vi "CloseConfigFP.vi"(8 "error in (no error)":errorcluster, 10 "Ancestor":string, 11 "reference in":refnum<class "ViPER.lvclass">) -> (0 "error out":errorcluster, 3 "reference out":refnum<class "ViPER.lvclass">)   [LabVIEW 2022 SP3, in "ViPER.lvlib" / "ViPER.lvclass"]
doc: "### BSD License (http://www.opensource.org/licenses/bsd-license.php) Begin ###\n\nCopyright (c) 2018 Kurt Friday www.medulla.net\n\nAll rights reserved.\n\nRedistribution and use in source and binary forms, with or without\nmodification, are permitted provided that the following conditions are met:\n\n * Redistributions of source code must retain the above copyright\n notice, this list of conditions and the following disclaimer.\n\n * Redistributions in binary form must reproduce the above copyright\n notice, this list of conditions and the following disclaimer in the\n documentation and/or other materials provided with the distribution.\n\n * Neither the name of the <organization> nor the\n names of its contributors may be used to endorse or promote products\n derived from this software without specific prior written permission.\n\nTHIS SOFTWARE IS PROVIDED BY THE COPYRIGHT HOLDERS AND CONTRIBUTORS \"AS IS\" AND\nANY EXPRESS OR IMPLIED WARRANTIES, INCLUDING, BUT NOT LIMITED TO, THE IMPLIED\nWARRANTIES OF MERCHANTABILITY AND FITNESS FOR A PARTICULAR PURPOSE ARE\nDISCLAIMED. IN NO EVENT SHALL <COPYRIGHT HOLDER> BE LIABLE FOR ANY\nDIRECT, INDIRECT, INCIDENTAL, SPECIAL, EXEMPLARY, OR CONSEQUENTIAL DAMAGES\n(INCLUDING, BUT NOT LIMITED TO, PROCUREMENT OF SUBSTITUTE GOODS OR SERVICES;\nLOSS OF USE, DATA, OR PROFITS; OR BUSINESS INTERRUPTION) HOWEVER CAUSED AND\nON ANY THEORY OF LIABILITY, WHETHER IN CONTRACT, STRICT LIABILITY, OR TORT\n(INCLUDING NEGLIGENCE OR OTHERWISE) ARISING IN ANY WAY OUT OF THE USE OF THIS\nSOFTWARE, EVEN IF ADVISED OF THE POSSIBILITY OF SUCH DAMAGE."
uses:
  ViPER.lvclass
panel:
  # "### BSD License (http://www.opensource.org/licenses/bsd-license.php) Begin ###\n\nCopyright (c) 2018  Kurt Friday www.medulla.net\n\nAll rights reserved.\n\nRedistribution and use in source and binary forms, with or without\nmodification, are permitted provided that the following conditions are met:\n\n    * Redistributions of source code must retain the above copyright\n      notice, this list of conditions and the following disclaimer.\n\n    * Redistributions in binary form must reproduce the above copyright\n      notice, this list of conditions and the following disclaimer in the\n      documentation and/or other materials provided with the distribution.\n\n    * Neither the name of the <organization> nor the\n      names of its contributors may be used to endorse or promote products\n      derived from this software without specific prior written permission.\n\nTHIS SOFTWARE IS PROVIDED BY THE COPYRIGHT HOLDERS AND CONTRIBUTORS \"AS IS\" AND\nANY EXPRESS OR IMPLIED WARRANTIES, INCLUDING, BUT NOT LIMITED TO, THE IMPLIED\nWARRANTIES OF MERCHANTABILITY AND FITNESS FOR A PARTICULAR PURPOSE ARE\nDISCLAIMED. IN NO EVENT SHALL <COPYRIGHT HOLDER> BE LIABLE FOR ANY\nDIRECT, INDIRECT, INCIDENTAL, SPECIAL, EXEMPLARY, OR CONSEQUENTIAL DAMAGES\n(INCLUDING, BUT NOT LIMITED TO, PROCUREMENT OF SUBSTITUTE GOODS OR SERVICES;\nLOSS OF USE, DATA, OR PROFITS; OR BUSINESS INTERRUPTION) HOWEVER CAUSED AND\nON ANY THEORY OF LIABILITY, WHETHER IN CONTRACT, STRICT LIABILITY, OR TORT\n(INCLUDING NEGLIGENCE OR OTHERWISE) ARISING IN ANY WAY OUT OF THE USE OF THIS\nSOFTWARE, EVEN IF ADVISED OF THE POSSIBILITY OF SUCH DAMAGE."
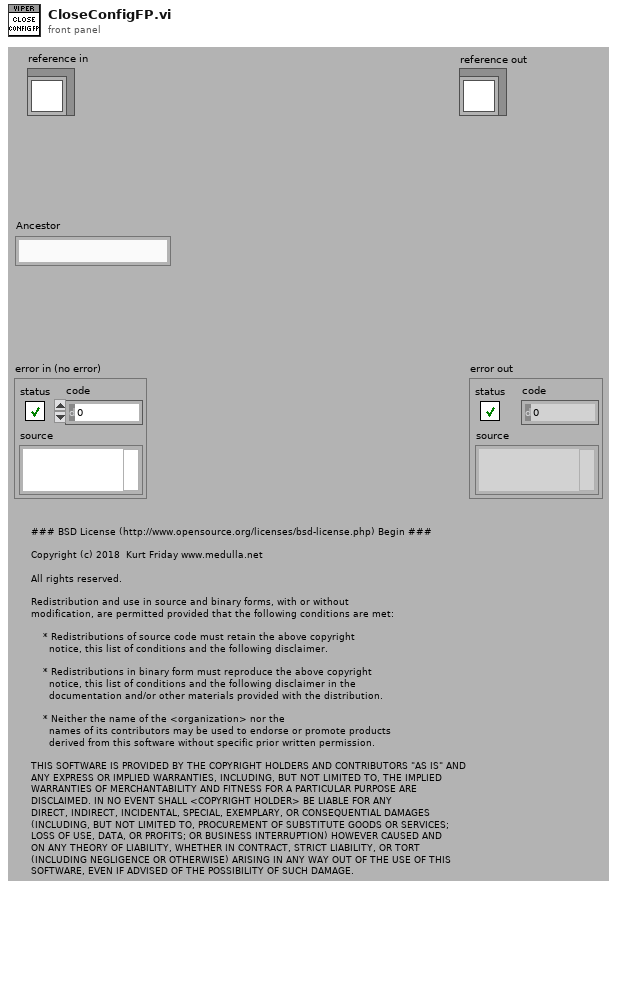
[diagram p1: front panel]
types:
  T1 = typedef "ViPER.lvlib/ViPER.lvclass/Details.ctl" = cluster{"Name":string, "Class":string}
  T2 = typedef "ViPER.lvlib/ViPER.lvclass/ObjectAttributes.ctl" = cluster{"Object":T3, "Ancestors":T5[], "Config":T6, "Init_OK":bool, "Hierachy":string[], "PPL?":bool[], "SFP_Open":bool[], "Config_SFP_Open":bool[], "SoftFP_event":refnum<user-event>[], "ConfigFP_event":refnum<user-event>[], "SoftFP_Shutdown_Notifier":refnum<notifier>[], "ConfigFP_Shutdown_Notifier":refnum<notifier>[]}
  T3 = typedef "ViPER.lvlib/ViPER.lvclass/ObjectDefinition.ctl" = cluster{"Name":string, "Ancestors":T4[]}
  T4 = typedef "ViPER.lvlib/ViPER.lvclass/Ancestor.ctl" = cluster{"Class":string, "Config":string, "Objects":string[]}
  T5 = typedef "ViPER.lvlib/ViPER.lvclass/ObjectLayers.ctl" = cluster{"Ancestor":string, "Objects":refnum<class "ViPER.lvclass">[], "Object_Names":string[], "Owned":bool[]}
  T6 = typedef "ViPER.lvlib/ViPER.lvclass/Config.ctl" = cluster{"default":string}
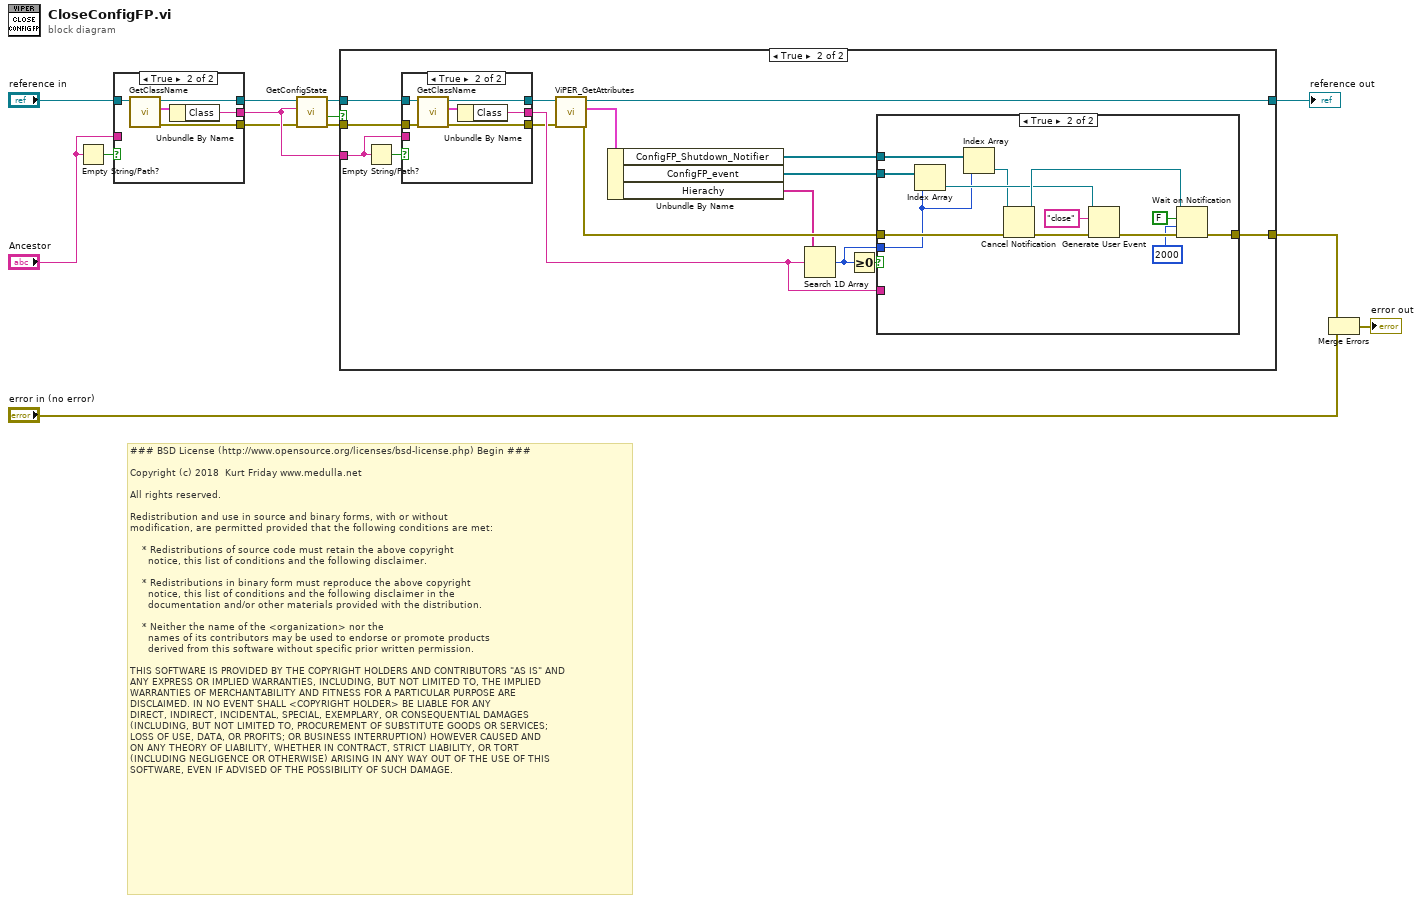
[diagram p0: block diagram]
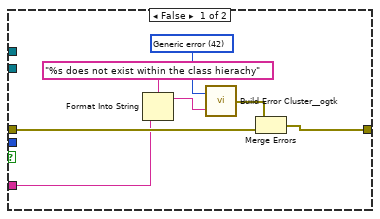
[diagram p5: hidden frame]
diagram:
  # "### BSD License (http://www.opensource.org/licenses/bsd-license.php) Begin ###\n\nCopyright (c) 2018  Kurt Friday www.medulla.net\n\nAll rights reserved.\n\nRedistribution and use in source and binary forms, with or without\nmodification, are permitted provided that the following conditions are met:\n\n    * Redistributions of source code must retain the above copyright\n      notice, this list of conditions and the following disclaimer.\n\n    * Redistributions in binary form must reproduce the above copyright\n      notice, this list of conditions and the following disclaimer in the\n      documentation and/or other materials provided with the distribution.\n\n    * Neither the name of the <organization> nor the\n      names of its contributors may be used to endorse or promote products\n      derived from this software without specific prior written permission.\n\nTHIS SOFTWARE IS PROVIDED BY THE COPYRIGHT HOLDERS AND CONTRIBUTORS \"AS IS\" AND\nANY EXPRESS OR IMPLIED WARRANTIES, INCLUDING, BUT NOT LIMITED TO, THE IMPLIED\nWARRANTIES OF MERCHANTABILITY AND FITNESS FOR A PARTICULAR PURPOSE ARE\nDISCLAIMED. IN NO EVENT SHALL <COPYRIGHT HOLDER> BE LIABLE FOR ANY\nDIRECT, INDIRECT, INCIDENTAL, SPECIAL, EXEMPLARY, OR CONSEQUENTIAL DAMAGES\n(INCLUDING, BUT NOT LIMITED TO, PROCUREMENT OF SUBSTITUTE GOODS OR SERVICES;\nLOSS OF USE, DATA, OR PROFITS; OR BUSINESS INTERRUPTION) HOWEVER CAUSED AND\nON ANY THEORY OF LIABILITY, WHETHER IN CONTRACT, STRICT LIABILITY, OR TORT\n(INCLUDING NEGLIGENCE OR OTHERWISE) ARISING IN ANY WAY OUT OF THE USE OF THIS\nSOFTWARE, EVEN IF ADVISED OF THE POSSIBILITY OF SUCH DAMAGE."
  n1 = Empty String/Path?(string/path="Ancestor") -> (empty?=w6:bool)
  n2 = case shown="True" w6 {
    tunnel: [_ w20] -> w1
    tunnel: "reference in" -> [w15 w19]
    tunnel: [w15 w18] -> w4
    tunnel: "Ancestor" -> [w14 _]
    tunnel: [w14 w16] -> w2
    frame False {
    }
    frame True {
      n3 = call "GetClassName.vi"("reference in"=w19) -> ("error out"=w20:errorcluster, "Details"=w17:T1, "reference out"=w18:refnum<class "ViPER.lvclass">)  [unwired: 8 in]
      n4 = Unbundle By Name(w17) -> ("Class"=w16:string)
    }
  }
  n5 = call-dynamic "GetConfigState.vi"("error in (no error)"=w1, "Ancestor"=w2, "reference in"=w4) -> ("error out"=w10:errorcluster, "config_open"=w9:bool, "reference out"=w11:refnum<class "ViPER.lvclass">)  [unwired: 6 in]
  n6 = case shown="True" w9 {
    tunnel: [w21 w36] -> w7
    tunnel: [w22 w35] -> w8
    tunnel: w11 -> [w22 w29]
    tunnel: w10 -> [w21 w27]
    tunnel: w2 -> [_ w24]
    frame False {
    }
    frame True {
      n7 = Empty String/Path?(string/path=w24) -> (empty?=w26:bool)
      n8 = case shown="True" w26 {
        tunnel: w27 -> [w39 w47]
        tunnel: [w39 w46] -> w23
        tunnel: w29 -> [w41 w45]
        tunnel: [w41 w44] -> w28
        tunnel: w24 -> [w40 _]
        tunnel: [w40 w42] -> w25
        frame False {
        }
        frame True {
          n9 = call "GetClassName.vi"("error in (no error)"=w47, "reference in"=w45) -> ("error out"=w46:errorcluster, "Details"=w43:T1, "reference out"=w44:refnum<class "ViPER.lvclass">)  [unwired: 7 in]
          n10 = Unbundle By Name(w43) -> ("Class"=w42:string)
        }
      }
      n11 = call "ViPER_GetAttributes.vi"("error in (no error)"=w23, "reference in"=w28) -> ("error out"=w34:errorcluster, "Data"=w38:T2, "reference out"=w35:refnum<class "ViPER.lvclass">)  [unwired: 6 in, 1 out]
      n12 = Unbundle By Name(w38) -> ("ConfigFP_Shutdown_Notifier"=w33:refnum<notifier>[], "ConfigFP_event"=w37:refnum<user-event>[], "Hierachy"=w32:string[])
      n13 = Search 1D Array(1D array=w32, element=w25) -> (index of element=w30:i32)  [unwired: 1 in]
      n14 = Greater Or Equal To 0?(x=w30) -> (x >= 0?=w31:bool)
      n15 = case shown="True" w31 {
        tunnel: w37 -> [_ w59]
        tunnel: [w49 w67] -> w36
        tunnel: w34 -> [w50 w66]
        tunnel: w33 -> [_ w57]
        tunnel: w30 -> [_ w56]
        tunnel: w25 -> [w48 _]
        frame False {
          w51 = 42 items=["No error", "Argument error", "Memory is full", "Out of zone", "End of file", "File already open", "Generic file I/O error", "File not found", "File permission error", "Disk is full", "Duplicate path", "Too many files open", "System feature not enabled", "Resource file not found", "Cannot add resource", "Resource not found", "Image not found", "Image memory error", "Pen does not exist", "Config type invalid", "Config token not found", "Config parse error", "Config memory error", "Bad external code format", "Bad external code offset", "External code not present", "Null window", "Destroy window error", "Null menu", "Print aborted", "Bad print record", "Print driver error", "Windows error during printing", "Memory error during printing", "Print dialog error", "Generic print error", "Invalid device refnum", "Device not found", "Device parameter error", "Device unit error", "Cannot open device", "Device call aborted", "Generic error", "Cancelled by user", "Object ID too low", "Object ID too high", "Object not in heap", "Unknown heap", "Unknown object (invalid DefProc)", "Unknown object (DefProc not in table)", "Message out of range", "Invalid (null) method", "Unknown message", "Manager call not supported", "Bad address", "Network operation in progress", "Network operation timed out", "Connection is busy", "Network attribute not supported", "Network error", "Address in use", "System out of memory", "Connection aborted", "Connection refused", "Not connected", "Already connected", "Connection closed", "Initialization error (interapplication manager)", "Bad occurrence", "Wait on unbound occurrence handler", "Occurrence queue overflow", "Datalog type conflict", "Unused", "Unrecognized type (interapplication manager)", "Memory corrupt", "Failed to make temporary DLL", "Old CIN version", "Drag socket not found", "Failed to load drop-object", "Failed to register OLE object", "Failed to release OLE object", "Format specifier type mismatch", "Unknown format specifier", "Too few format specifiers", "Too many format specifiers", "Scan failed", "Newer CIN version", "Error converting to variant", "Runtime menu error", "Password tampered", "Variant attribute not found", "Incompatible variant data type", "Event data is not available", "Event Store is not present", "Occurrence is not found", "Event Queue is not created", "Event info is not available", "Refnum passed is NULL", "Error retrieving Class GUID", "Error retrieving CoClass GUID", "Error retrieving TypeLib GUID.", "Bad built application magic bytes.", "Specific driver is different from the specific driver associated with the Logical Name.", "There is no session opened to the class driver.", "Max Error", "MAX - Error with config objects", "MAX - Error loading configuration", "MAX - Group not supported"]
          n16 = Format Into String(format string="%s does not exist within the class hierachy", w48) -> (resulting string=w54:string)  [unwired: 2 in, 1 out]
          n17 = call <userlib>:"Build Error Cluster__ogtk.vi"("String to Prepend to source (\"\")"=w54, "code"=w51) -> ("error out"=w52:errorcluster)
          n18 = Merge Errors(w52, w50) -> (w49:errorcluster)
        }
        frame True {
          n19 = Index Array(array=w59, index=w56) -> (element=w58:refnum<user-event>)
          n20 = Index Array(array=w57, index=w56) -> (element=w55:refnum<notifier>)
          n21 = Cancel Notification(0:w55, 3:w66) -> (8:w64:refnum<notifier>, 11:w65:errorcluster)  [unwired: 1 out]
          n22 = Generate User Event(user event=w58, event data cluster="close" ("event data"), error in=w65) -> (error out=w62:errorcluster)  [unwired: 1 in, 1 out]
          n23 = Wait on Notification(notifier=w64, ignore previous (F)=FALSE, timeout in ms (-1)=2000, error in (no error)=w62) -> (error out=w67:errorcluster)  [unwired: 3 out]
        }
      }
    }
  }
  "reference out" <- w8
  n24 = Merge Errors(w7, "error in (no error)") -> (→"error out":errorcluster)
